vi "RSNRPZ Configure Scope.vi"(0 "VISA session":refnum<visa-resource-name> caption="VISA resource name", 1 "Offset Time (0.0 s)":dbl format="%.2p", 5 "Channel (1)":i32=1, 7 "Scope Points (312)":i32=312, 9 "Scope Time (0.01 s)":dbl=0.01 format="%.2p", 11 "error in (no error)":errorcluster, 12 "Realtime (F: Off)":bool) -> (4 "dup VISA session":refnum<visa-resource-name> caption="VISA resource name", 15 "error out":errorcluster)   [LabVIEW 2010]
doc: "This VI sets parameters of the Scope mode.\n\nNote:\n\n1) This VI is not available for NRP-Z51.\n\nRemote-control command(s):\nSENS:TRAC:POIN\nSENS:TRAC:TIME\nSENS:TRAC:OFFS:TIME\nSENS:TRAC:REAL ON | OFF"
uses:
  rsnrpz_32.dll
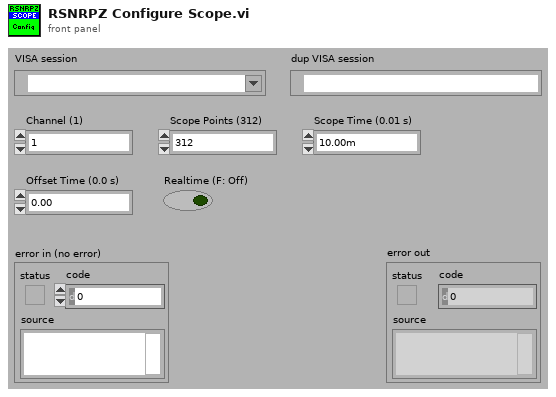
[diagram p1: front panel]
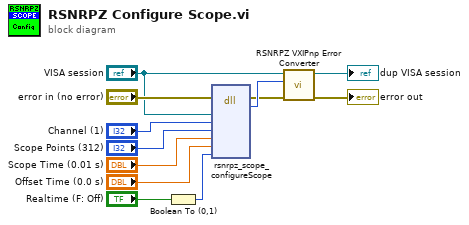
[diagram p0: block diagram]
diagram:
  n1 = Boolean To (0,1)(Boolean="Realtime (F: Off)") -> (0, 1=w6:i16)
  n2 = dll-call lib="rsnrpz_32.dll" fn="rsnrpz_scope_configureScope"(error in="error in (no error)", "VISA Session"="VISA session", "Channel"="Channel (1)", "Scope Points"="Scope Points (312)", "Scope Time"="Scope Time (0.01 s)", "Offset Time"="Offset Time (0.0 s)", "Realtime"=w6) -> (error out=w5:errorcluster, "Status"=w11:i32)  [unwired: 8 in, 1 out]
  n3 = call <instrlib>:"RSNRPZ VXIPnp Error Converter.vi"("error in"=w5, "VXIPnp error code"=w11, "VISA session"="VISA session") -> ("error out"=→"error out":errorcluster, "dup VISA session"=→"dup VISA session":refnum<visa-resource-name>)  [unwired: 7 in]
